vi "Set_Autotest Ok _.vi"(8 "error in (no error)":errorcluster caption="entrée d'erreur (pas d'erreur)", 10 "Autotest Ok ?":bool, 11 "Class Instrument (Default) en entrée":refnum<class "Class Instrument (Default).lvclass">) -> (0 "error out":errorcluster caption="sortie d'erreur", 3 "Class Instrument (Default) en sortie":refnum<class "Class Instrument (Default).lvclass">)   [LabVIEW 2020, in "Library Instrument & Equipement.lvlib" / "Library Instruments.lvlib" / "Class Instrument (Default).lvclass"]
uses:
  Class Instrument (Default).lvclass
  Class Instrument (Default).lvclass/Class Instrument (Default).ctl
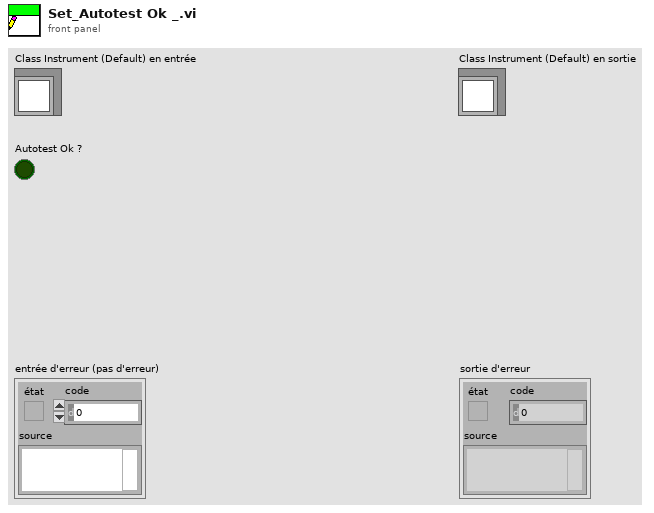
[diagram p1: front panel]
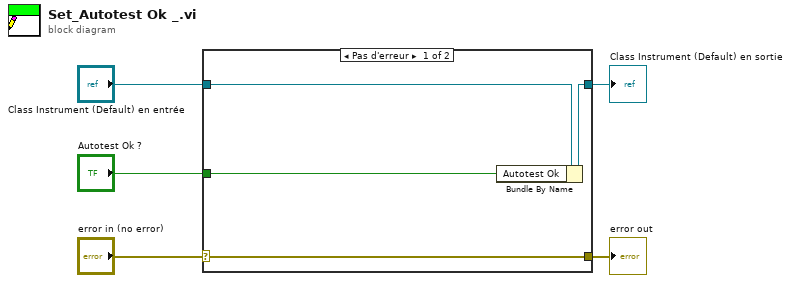
[diagram p0: block diagram]
diagram:
  n1 = case shown="Pas d'erreur" "error in (no error)" {
    selector: "error in (no error)" -> [w9 w10]
    tunnel: [w9 w10] -> w4
    tunnel: [w7 w11] -> w2
    tunnel: "Class Instrument (Default) en entrée" -> [w8 w11]
    tunnel: "Autotest Ok ?" -> [w6 _]
    frame No Error {
      n2 = Bundle By Name(cluster=w8, "Autotest Ok"=w6) -> (w7:refnum<class "Class Instrument (Default).lvclass">)
    }
    frame Error {
    }
  }
  "error out" <- w4
  "Class Instrument (Default) en sortie" <- w2
